vi "PlaySound.vi"(8 "error in (no error)":errorcluster, 9 "Overwrite":bool, 10 "Name":string, 11 "Game in":refnum<class "Game.lvclass">) -> (0 "error out":errorcluster, 3 "Game out":refnum<class "Game.lvclass">)   [LabVIEW 2019, in "RT_Game.lvlib" / "Game.lvclass"]
uses:
  Game.lvclass
  Engine/MessageCluster.ctl
  Engine/PlaySoundData.ctl
  Game.lvclass/Game.ctl
  Engine/Engine.lvclass
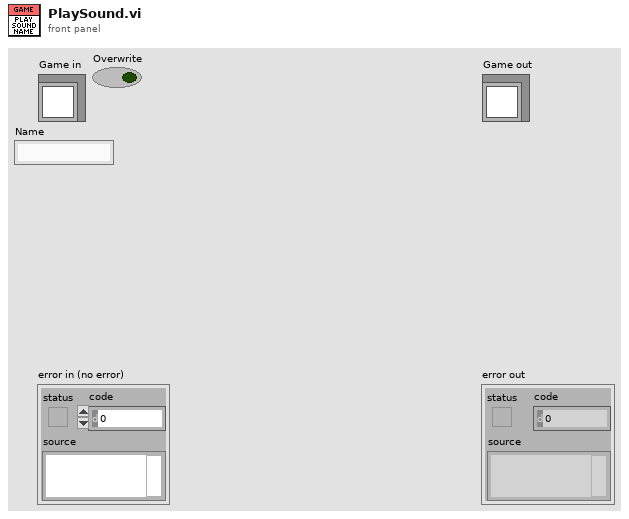
[diagram p1: front panel]
types:
  T1 = typedef "RT_Game.lvlib/Engine.lvclass/PlaySoundData.ctl" = cluster{"Name":string, "Overwrite":bool}
  T2 = typedef "RT_Game.lvlib/Engine.lvclass/MessageCluster.ctl" = cluster{"Message":string, "Data":variant}
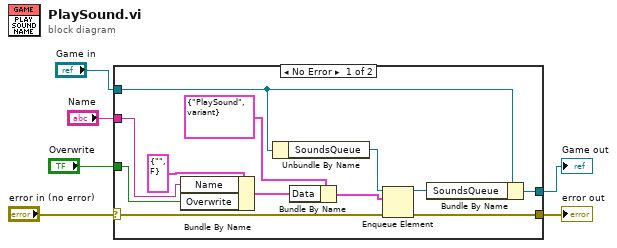
[diagram p0: block diagram]
diagram:
  n1 = case shown="No Error" "error in (no error)" {
    selector: "error in (no error)" -> [w18 w20]
    tunnel: [w17 w20] -> w5
    tunnel: [w14 w19] -> w3
    tunnel: "Game in" -> [w16 w19]
    tunnel: "Overwrite" -> [w8 _]
    tunnel: "Name" -> [w7 _]
    frame No Error {
      n2 = Bundle By Name(cluster=T1 {"Name"="", "Overwrite"=FALSE} ("PlaySoundData"), "Name"=w7, "Overwrite"=w8) -> (w9:T1)
      n3 = Unbundle By Name(w16) -> ("SoundsQueue"=w15:refnum<queue>)
      n4 = Bundle By Name(cluster=T2 {"Message"="PlaySound", "Data"=variant} ("element"), "Data"=w9) -> (w11:T2)
      n5 = Enqueue Element(queue=w15, element=w11, error in (no error)=w18) -> (queue out=w13:refnum<queue>, error out=w17:errorcluster)  [unwired: 1 in, 1 out]
      n6 = Bundle By Name(cluster=w16, "SoundsQueue"=w13) -> (w14:refnum<class "Game.lvclass">)
    }
    frame Error {
    }
  }
  "error out" <- w5
  "Game out" <- w3
